vi "HackRF_Demod(SubVI).vi"(11 "Read":u8[](array[numeric])) -> (3 "dX/dt":dbl[](array[numeric]))   [LabVIEW 2013]
uses:
  <vilib>/Analysis/3filter.llb/Elliptic Filter (DBL).vi
  <vilib>/Analysis/NI_AALBase.lvlib
  <vilib>/Analysis/NI_AALPro.lvlib
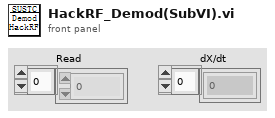
[diagram p1: front panel]
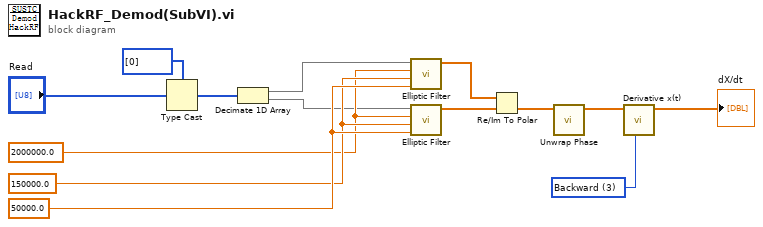
[diagram p0: block diagram]
diagram:
  w12 = u16 3 items=["2nd Order Central", "4th Order Central", "Forward", "Backward"] ("method")
  w9 = 50000.0 ("low cutoff freq: fl")
  w8 = 150000.0 ("high cutoff freq: fh")
  w7 = 2000000.0 ("sampling freq: fs")
  n1 = Type Cast(type=i8[] [0] ("Read"), x="Read") -> (*(type *) &x=w3:i8[])
  n2 = Decimate 1D Array(w3) -> (w6:i8[], w4:i8[])
  n3 = call-poly <vilib>:"Elliptic Filter.vi"("low cutoff freq: fl"=w9, "high cutoff freq: fh"=w8, "sampling freq: fs"=w7, "X"=w6) -> ("Filtered X"=w1:dbl[])  [unwired: 6 in, 1 out]
  n4 = call-poly <vilib>:"Elliptic Filter.vi"("low cutoff freq: fl"=w9, "high cutoff freq: fh"=w8, "sampling freq: fs"=w7, "X"=w4) -> ("Filtered X"=w5:dbl[])  [unwired: 6 in, 1 out]
  n5 = Re/Im To Polar(2:w5, 3:w1) -> (0:w13:dbl[])  [unwired: 1 out]
  n6 = call <vilib>:"Unwrap Phase.vi"("Phase"=w13) -> ("Unwrapped Phase"=w11:dbl[])  [unwired: 9 in, 1 out]
  n7 = call <vilib>:"Derivative x(t).vi"("method"=w12, "X"=w11) -> ("dX/dt"=→"dX/dt":dbl[])  [unwired: 8 in, 1 out]
